vi "LoadCoeffsFromEprom.vi"(8 "error in":errorcluster, 11 "StellarNetSpectrometer in":refnum<class "StellarNetSpectrometer.lvclass">) -> (0 "error out":errorcluster, 3 "StellarNetSpectrometer out":refnum<class "StellarNetSpectrometer.lvclass">)   [LabVIEW 2013, in "StellarNetSpectrometer.lvclass"]
doc: "Read the Coefficients and the Detector Specifier from the device EEPROM"
uses:
  StellarNetSpectrometer.lvclass
  StellarNetSpectrometer.lvclass/StellarNetSpectrometer.ctl
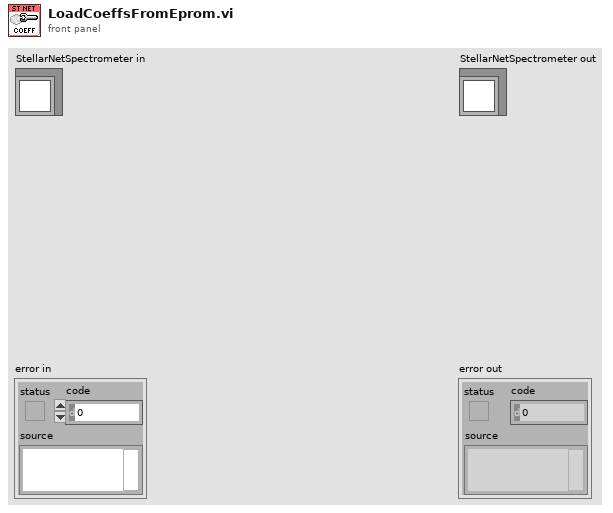
[diagram p1: front panel]
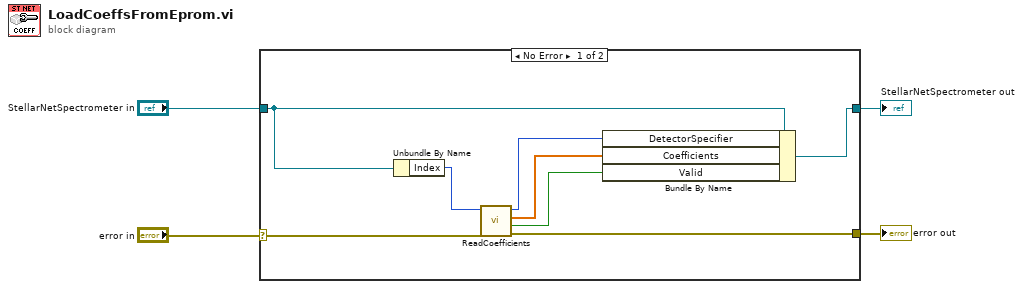
[diagram p0: block diagram]
diagram:
  n1 = case shown="No Error" "error in" {
    selector: "error in" -> [w12 w14]
    tunnel: [w11 w14] -> w3
    tunnel: [w6 w13] -> w1
    tunnel: "StellarNetSpectrometer in" -> [w10 w13]
    frame No Error {
      n2 = Unbundle By Name(w10) -> ("Index"=w5:u32)
      n3 = call "ReadCoefficients.vi"("error in"=w12, "Channel(1)"=w5) -> ("error out"=w11:errorcluster, "Valid"=w8:bool, "Coefficients"=w9:ext[], "SelectorSpecifier"=w7:u16)  [unwired: 6 in]
      n4 = Bundle By Name(cluster=w10, "DetectorSpecifier"=w7, "Coefficients"=w9, "Valid"=w8) -> (w6:refnum<class "StellarNetSpectrometer.lvclass">)
    }
    frame Error {
    }
  }
  "error out" <- w3
  "StellarNetSpectrometer out" <- w1
